vi "I2C Write Register (16bit).vi"(7 "MSB(yte) First? (F=Lo->Hi)":bool, 8 "error in (no error)":errorcluster, 9 "Value":u16, 10 "Register Address":u8, 11 "LINX I2C in":refnum<class "LINX I2C.lvclass">) -> (0 "error out":errorcluster, 3 "LINX I2C out":refnum<class "LINX I2C.lvclass">)   [LabVIEW 2020, in "LINX I2C.lvclass"]
doc: "Writes a 16-bit value to the register address."
uses:
  LINX I2C.lvclass
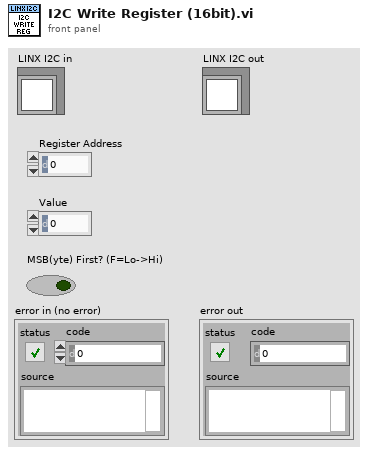
[diagram p1: front panel]
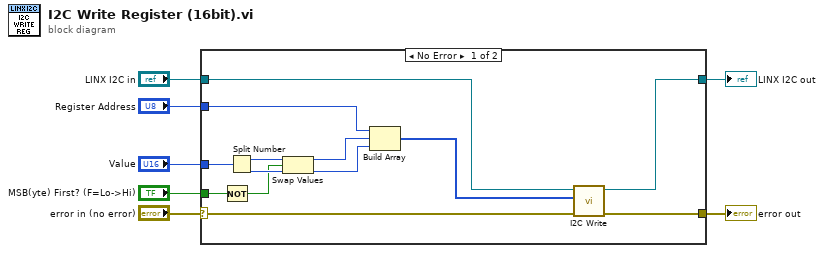
[diagram p0: block diagram]
diagram:
  n1 = case shown="No Error" "error in (no error)" {
    selector: "error in (no error)" -> [w18 w21]
    tunnel: [w19 w22] -> w7
    tunnel: "LINX I2C in" -> [w20 w22]
    tunnel: [w17 w21] -> w5
    tunnel: "Register Address" -> [w16 _]
    tunnel: "Value" -> [w15 _]
    tunnel: "MSB(yte) First? (F=Lo->Hi)" -> [w11 _]
    frame No Error {
      n2 = Not(x=w11) -> (.not. x?=w8:bool)
      n3 = Split Number(x=w15) -> (hi(x)=w13:u8, lo(x)=w12:u8)
      n4 = Swap Values(12:w13, 13:w8, 14:w12) -> (1:w10:u8, 3:w9:u8)
      n5 = Build Array(w16, w10, w9) -> (w14:u8[])
      n6 = call "I2C Write.vi"("error in (no error)"=w18, "Bytes to Write"=w14, "LINX I2C in"=w20) -> ("error out"=w17:errorcluster, "LINX I2C out"=w19:refnum<class "LINX I2C.lvclass">)  [unwired: 7 in]
    }
    frame Error {
    }
  }
  "LINX I2C out" <- w7
  "error out" <- w5
